vi "Set Bucket Website.vi"(8 "error in (no error)":errorcluster, 10 "Website Configuration":T1, 11 "Bucket in":refnum<class "Bucket.lvclass">) -> (0 "error out":errorcluster, 3 "Bucket out":refnum<class "Bucket.lvclass">)   [LabVIEW 2015, in "NI_AWS_S3.lvlib" / "Bucket.lvclass"]
doc: "Sets the configuration of the website that is specified in the website subresource. To configure a bucket as a website, you can add this subresource on the bucket with website configuration information such as the file name of the index document and any redirect rules."
uses:
  Bucket.lvclass
  Website Configuration.ctl
  Core/HTTP Request/Region handling.ctl
  Core/HTTP Request/Name Value Pair.ctl
  Core/HTTP Request/Request Options.ctl
  Core/HTTP Request/URL formatting.ctl
  Bucket.lvclass/Bucket.ctl
  Read Name.vi
  Core/HTTP Request/HTTP Request.lvclass
  NI_AWS_S3.lvlib
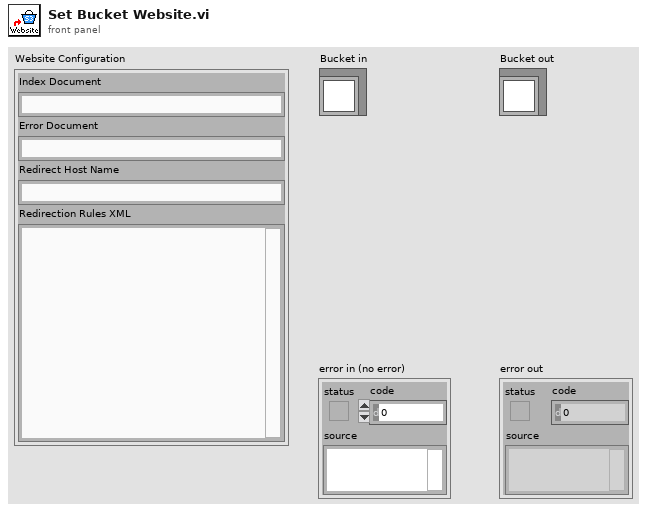
[diagram p1: front panel]
types:
  T1 = typedef "NI_AWS_S3.lvlib/Website Configuration.ctl" = cluster{"Index Document":string, "Error Document":string, "Redirect Host Name":string, "Redirection Rules XML":string}
  T2 = typedef "NI_AWS_Core.lvlib/HTTP Request.lvclass/Request Options.ctl" = cluster{"request headers":T3[], "request parameters":T3[], "request body":string, "region handling":T4, "URL formatting":T5}
  T3 = typedef "NI_AWS_Core.lvlib/HTTP Request.lvclass/Name Value Pair.ctl" = cluster{"name":string, "value":string}
  T4 = typedef "NI_AWS_Core.lvlib/HTTP Request.lvclass/Region handling.ctl" = enum16{"use region everywhere", "use region (authentication only)", "use region (URL only)", "ignore region everwhere"}
  T5 = typedef "NI_AWS_Core.lvlib/HTTP Request.lvclass/URL formatting.ctl" = enum16{"region-", "region."}
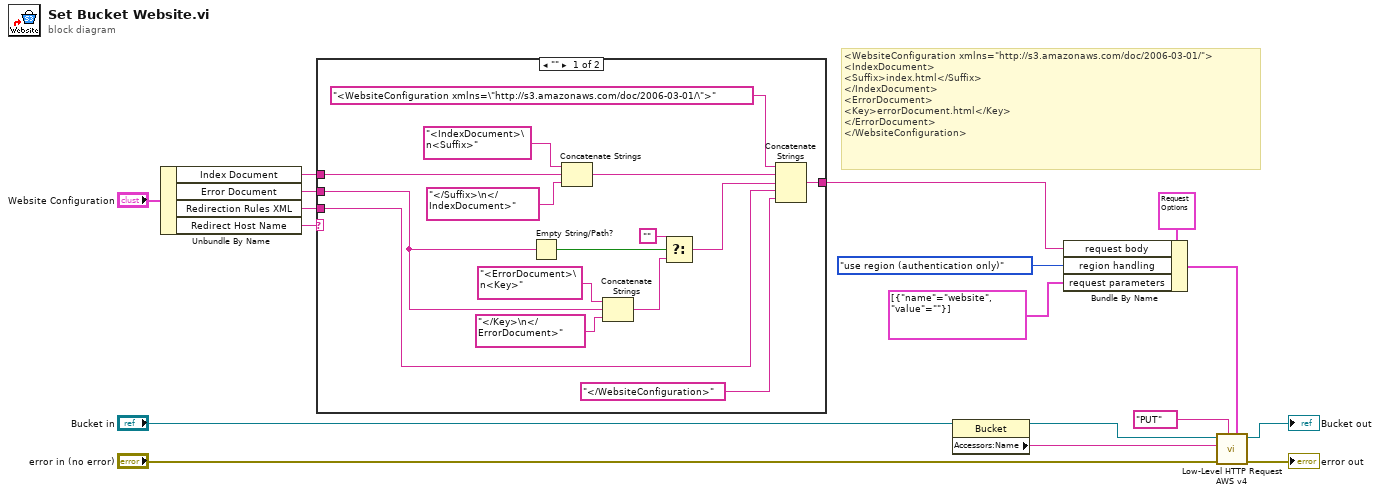
[diagram p0: block diagram]
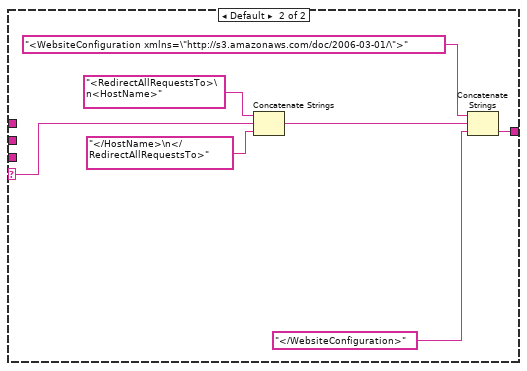
[diagram p2: hidden frame]
diagram:
  # "<WebsiteConfiguration xmlns=\"http://s3.amazonaws.com/doc/2006-03-01/\">\n<IndexDocument>\n<Suffix>index.html</Suffix>\n</IndexDocument>\n<ErrorDocument>\n<Key>errorDocument.html</Key>\n</ErrorDocument>\n</WebsiteConfiguration>"
  n1 = Unbundle By Name("Website Configuration") -> ("Index Document"=w6:string, "Error Document"=w5:string, "Redirection Rules XML"=w3:string, "Redirect Host Name"=w4:string)
  n2 = case shown="\"\"" w4 {
    selector: w4 -> [_ w33]
    tunnel: w6 -> [w31 _]
    tunnel: [w21 w35] -> w1
    tunnel: w5 -> [w20 _]
    tunnel: w3 -> [w18 _]
    frame "" {
      n3 = Empty String/Path?(string/path=w20) -> (empty?=w27:bool)
      n4 = Concatenate Strings("<IndexDocument>\n<Suffix>", w31, "</Suffix>\n</IndexDocument>") -> (w23:string)
      n5 = Concatenate Strings("<ErrorDocument>\n<Key>", w20, "</Key>\n</ErrorDocument>") -> (w26:string)
      n6 = Select(t="", s=w27, f=w26) -> (s? t:f=w22:string)
      n7 = Concatenate Strings("<WebsiteConfiguration xmlns=\"http://s3.amazonaws.com/doc/2006-03-01/\">", w23, w22, w18, "</WebsiteConfiguration>") -> (w21:string)
    }
    frame Default {
      n8 = Concatenate Strings("<RedirectAllRequestsTo>\n<HostName>", w33, "</HostName>\n</RedirectAllRequestsTo>") -> (w36:string)
      n9 = Concatenate Strings("<WebsiteConfiguration xmlns=\"http://s3.amazonaws.com/doc/2006-03-01/\">", w36, "</WebsiteConfiguration>") -> (w35:string)
    }
  }
  n10 = property class="Bucket"(reference="Bucket in") -> (reference out=w7:refnum<class "Bucket.lvclass">, "Accessors:Name"=w13:string)  [unwired: 1 in, 1 out]
  n11 = Bundle By Name(cluster=T2 {"request headers"=[], "request parameters"=[], "request body"="", "region handling"=enum."use region everywhere", "URL formatting"=enum."region."} ("Request Options"), "request body"=w1, "region handling"=Region_handling."use region (authentication only)", "request parameters"=T3[] [{"name"="website", "value"=""}]) -> (w8:T2)
  n12 = call "Low-Level HTTP Request AWS v4.vi"("Request Options"=w8, "HTTP-Verb"="PUT", "error in (no error)"="error in (no error)", "URL Prefix"=w13, "AWS Core in"=w7) -> ("error out"=→"error out":errorcluster, "AWS Core out"=→"Bucket out":refnum<class "Bucket.lvclass">)  [unwired: 3 in, 2 out]
